vi "Pump Start Detector (Kuhnke).vi"(6 "Reset":bool, 9 "Pos?":bool, 10 "Window":i32, 11 "Pos Cross":bool) -> (1 "Spikes":i32, 3 "Starts":u32)   [LabVIEW 2019]
uses:
  <vilib>/Platform/TimedLoop/XDataNode/timing_clust.ctl
  <vilib>/Platform/TimedLoop/XDataNode/nitl_modes.ctl
  <vilib>/Platform/TimedLoop/XDataNode/wakeup.ctl
  <vilib>/rvi/Emulation/niFpgaSctlEmulationGetInTimedLoop.vi
  <vilib>/rvi/Emulation/niFpgaEmulationReportErrorSimple.vi
  <vilib>/rvi/Emulation/niFpgaGetClockAttributes.vi
  <vilib>/rvi/Emulation/niFpgaCriticalErrorInLSC.vi
  <vilib>/Platform/TimedLoop/XDataNode/XDataNode.xnode
  <vilib>/Platform/TimedLoop/XDataNode/XDNodeRunTimeDep.lvlib
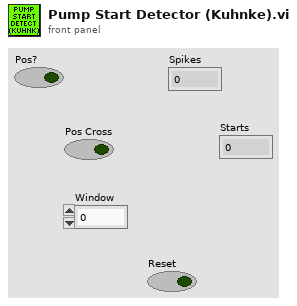
[diagram p1: front panel]
types:
  T1 = typedef "XDNodeRunTimeDep.lvlib/timing_clust.ctl" = cluster{"Expected End [f-1]":u64, "Actual End [f-1]":u64, "Finished Late? [f-1]":bool, "Expected End [i-1]":u64, "Actual End [i-1]":u64, "Finished Late? [i-1]":bool, "Expected Start [i]":u64, "Actual Start [i]":u64, "Expected Start [f]":u64, "Actual Start [f]":u64, "Source Name":string, "Structure Name":string, "Period":i64, "Deadline":i64, "Offset":i64, "Start":i64, "Priority":i32, "Timeout":i32, "Mode":T2, "Wakeup Reason":T3, "Error":errorcluster, "Source Type":string, "Secondary Source Type":string, "Global End Time":u64, "Global Start Time":u64, "Frame Duration":u64, "Iteration Duration":u64, "Assigned CPU":i32, "I/O Scan Engine Mode":u32}
  T2 = typedef "XDNodeRunTimeDep.lvlib/nitl_modes.ctl" = enum32{"No Change", "Process missed periods, maintain original phase", "Discard missed periods, maintain original phase", "Process missed periods, ignore original phase", "Discard missed periods, ignore original phase"}
  T3 = typedef "XDNodeRunTimeDep.lvlib/wakeup.ctl" = enum32{"Normal", "Aborted", "Asynchronous wakeup", "Timing source error", "Timed loop error", "Timeout"}
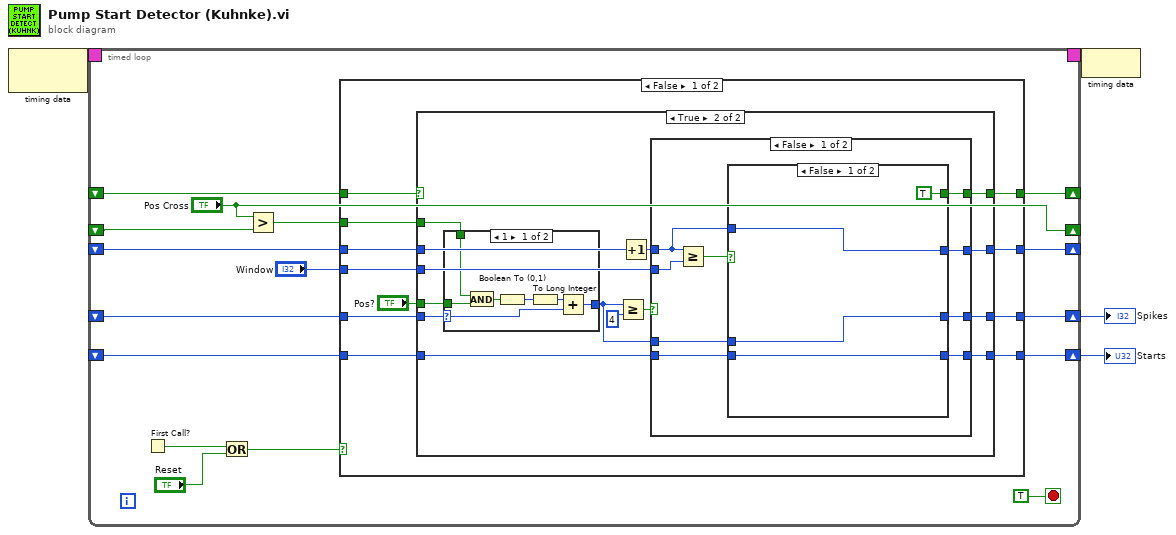
[diagram p0: block diagram]
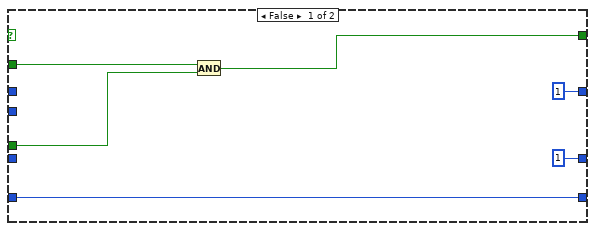
[diagram p2: hidden frame]
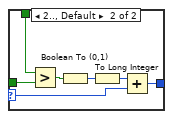
[diagram p3: hidden frame]
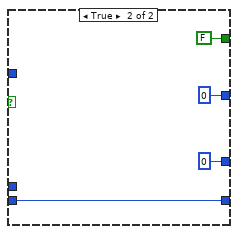
[diagram p4: hidden frame]
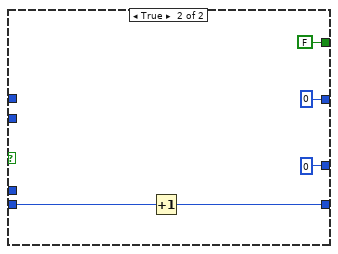
[diagram p5: hidden frame]
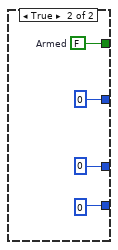
[diagram p6: hidden frame]
diagram:
  n1 = node-c288() -> (w4:T1)  [unwired: 1 in]
  n2 = timed-loop {
    shift-right: [w14] -> w2
    shift-left: _ -> [w15]
    shift-right: [w19] -> _
    shift-left: _ -> [w20]
    shift-right: [w18] -> _
    shift-left: _ -> [w17]
    timing: w4 -> [_]
    timing-out: [_] -> w3
    shift-right: ["Pos Cross"] -> _
    shift-left: _ -> [w6]
    shift-right: [w10] -> w1
    shift-left: _ -> [w9]
    stop <- TRUE stop-if-true
    n3 = First Call?() -> (First Call?: T/F=w13:bool)
    n4 = Or(x=w13, y="Reset") -> (x .or. y?=w12:bool)
    n5 = Greater?(x="Pos Cross", y=w6) -> (0:w5:bool)
    n6 = case shown="False" w12 {
      tunnel: w20 -> [w31 _]
      tunnel: [w30 w89] -> w19
      tunnel: [w28 0] -> w18
      tunnel: w17 -> [w26 _]
      tunnel: w15 -> [w24 _]
      tunnel: [w23 u32 0] -> w14
      tunnel: "Window" -> [w22 _]
      tunnel: w5 -> [w29 _]
      tunnel: [w27 0] -> w10
      tunnel: w9 -> [w25 _]
      frame False {
        n7 = case shown="True" w31 {
          tunnel: [w32 w44] -> w30
          tunnel: w29 -> [w33 w50]
          tunnel: [1 ("Window") w43] -> w28
          tunnel: [1 ("Window") w45] -> w27
          tunnel: w26 -> [_ w51]
          tunnel: w25 -> [_ w39]
          tunnel: w24 -> [w35 w47]
          tunnel: [w35 w46] -> w23
          tunnel: w22 -> [_ w41]
          tunnel: "Pos?" -> [w34 w38]
          frame False {
            n8 = And(x=w33, y=w34) -> (x .and. y?=w32:bool)
          }
          frame True {
            n9 = case shown="1" w39 {
              selector: w39 -> [w55 w59]
              tunnel: w50 -> [w54 w61]
              tunnel: [w57 w63] -> w40
              tunnel: w38 -> [w53 w62]
              frame 1 {
                n10 = And(x=w54, y=w53) -> (x .and. y?=w52:bool)
                n11 = Boolean To (0,1)(Boolean=w52) -> (0, 1=w58:i16)
                n12 = To Long Integer(number=w58) -> (32bit integer=w56:i32)
                n13 = Add(x=w56, y=w55) -> (x+y=w57:i32)
              }
              frame 2.., Default {
                n14 = Greater?(x=w61, y=w62) -> (0:w60:bool)
                n15 = Boolean To (0,1)(Boolean=w60) -> (0, 1=w65:i16)
                n16 = To Long Integer(number=w65) -> (32bit integer=w64:i32)
                n17 = Add(x=w64, y=w59) -> (x+y=w63:i32)
              }
            }
            n18 = Greater Or Equal?(x=w40, y=4) -> (x >= y?=w48:bool)
            n19 = Increment(x=w51) -> (x+1=w42:i32)
            n20 = case shown="False" w48 {
              tunnel: w47 -> [w72 w87]
              tunnel: [w71 w86] -> w46
              tunnel: [w70 0 ("Window")] -> w45
              tunnel: [w68 FALSE] -> w44
              tunnel: [w69 0 ("Window")] -> w43
              tunnel: w42 -> [w67 _]
              tunnel: w41 -> [w74 _]
              tunnel: w40 -> [w66 _]
              frame False {
                n21 = Greater Or Equal?(x=w67, y=w74) -> (x >= y?=w73:bool)
                n22 = case shown="False" w73 {
                  tunnel: [w78 w82] -> w71
                  tunnel: w72 -> [w78 w82]
                  tunnel: [w75 0 ("Window")] -> w70
                  tunnel: [w77 0 ("Window")] -> w69
                  tunnel: [TRUE FALSE] -> w68
                  tunnel: w67 -> [w77 _]
                  tunnel: w66 -> [w75 _]
                  frame False {
                  }
                  frame True {
                  }
                }
              }
              frame True {
                n23 = Increment(x=w87) -> (x+1=w86:u32)
              }
            }
          }
        }
      }
      frame True {
        w89 = FALSE  # Armed
      }
    }
  }
  "Starts" <- w2
  "Spikes" <- w1
  n24 = node-c288(w3) -> ()
